vi "PID % to EGU (DBL).vi"(1 "coerce output to range? (T)":bool=TRUE, 2 "minimum (EGU)":dbl format="%.2f", 3 "% span":dbl format="%.2f", 4 "maximum (EGU)":dbl format="%.2f") -> (0 "output (EGU)":dbl format="%.2f")   [LabVIEW 2020, in "NI_PID_pid.lvlib"]
doc: "Converts percent of range input to engineering-units output based upon the min & max range settings. The output is normally limited to the range [max...min]. Values outside of the range [max..min] are allowed when the input coerce output to range? (T) is FALSE."
uses:
  NI_PID_pid.lvlib
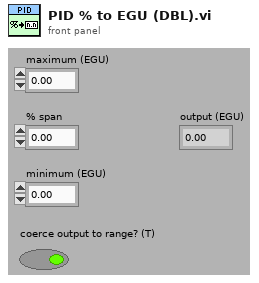
[diagram p1: front panel]
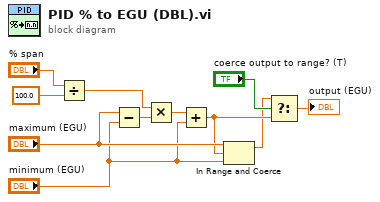
[diagram p0: block diagram]
diagram:
  n1 = Divide(x="% span", y=100.0) -> (x/y=w7:dbl)
  n2 = Subtract(x="maximum (EGU)", y="minimum (EGU)") -> (x-y=w11:dbl)
  n3 = Multiply(x=w7, y=w11) -> (x*y=w10:dbl)
  n4 = Add(x=w10, y="minimum (EGU)") -> (x+y=w3:dbl)
  n5 = In Range and Coerce(upper limit="maximum (EGU)", x=w3, lower limit="minimum (EGU)") -> (coerced(x)=w2:dbl)  [unwired: 1 out]
  n6 = Select(t=w2, s="coerce output to range? (T)", f=w3) -> (s? t:f=→"output (EGU)":dbl)
